vi "Calculate And Insert Biometry State.vi"(8 "error in (no error)":errorcluster caption="错误输入（无错误）", 10 "Measure_No":i64, 11 "connection reference":T1) -> (0 "error out":errorcluster caption="错误输出")   [LabVIEW 2015, in "Boimetry Processing.lvlib"]
doc: "对当初测量第几次的所有测试结果进行判断是否正常。\n判断的结果添加到Biometry的State数据库。\n输入：测量的第几次。"
uses:
  Boimetry Processing.lvlib
  <vilib>/addons/database/Connection.llb/Conn ObjectReference.ctl
  Database Processing/Support/Table/Biometry State.ctl
  Database Processing/Database Processing.lvlib
  <vilib>/addons/database/NI_Database_API.lvlib
  <vilib>/Analysis/NI_AALBase.lvlib
panel:
  # "Busy"
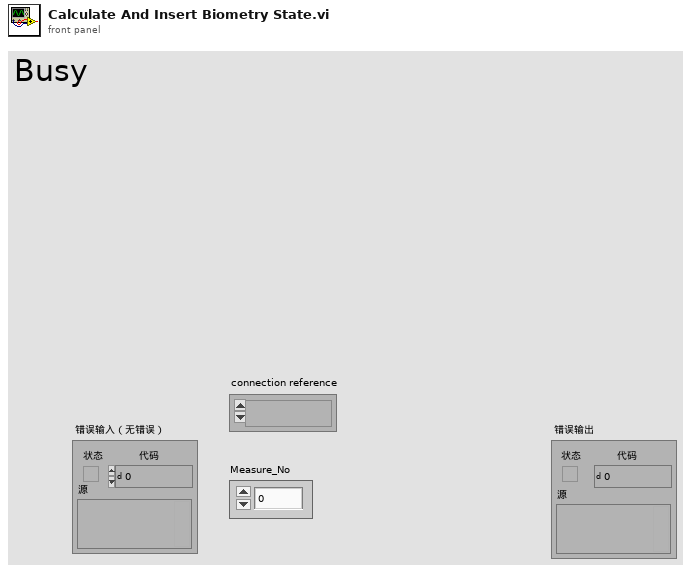
[diagram p1: front panel]
types:
  T1 = typedef "NI_Database_API.lvlib/Conn ObjectReference.ctl" = refnum<k1>
  T2 = typedef "Database Processing.lvlib/Biometry State.ctl" = cluster{"Measure_ID":i64, "Central_Corneal_Thickness_State":string, "Anterior_Chamber_Depth_State":string, "Len_Thickness_State":string, "Retinal_Thickness_State":string, "Axis_Length_State":string, "Pupil_Diameter_State":string, "White_To_White_State":string, "Keratometric_flat_State":string, "Keratometric_steep_State":string}
  T3 = typedef "Database Processing.lvlib/Biometry Attribute.ctl" = cluster{"Measure_ID":i64, "Measure_No":i64, "Ordinal":i64, "L_Or_R":string}
  T4 = typedef "Database Processing.lvlib/Biometry Parameter.ctl" = cluster{"Measure_ID":i64, "Central_Corneal_Thickness":sgl, "Anterior_Chamber_Depth":sgl, "Len_Thickness":sgl, "Retinal_Thickness":sgl, "Axis_Length":sgl, "Pupil_Diameter":sgl, "PCX":sgl, "PCY":sgl, "White_To_White":sgl, "ICX":sgl, "ICY":sgl, "Keratometric_flat":sgl, "Keratometric_steep":sgl, "Keratometric_Axis(flat)":sgl, "Keratometric_Axis(steep)":sgl, "Keratometric_AST":sgl}
  T5 = typedef "Boimetry Processing.lvlib/Limit Configuration.ctl" = cluster{"上限":dbl, "下限":dbl, "误差范围":dbl}[]
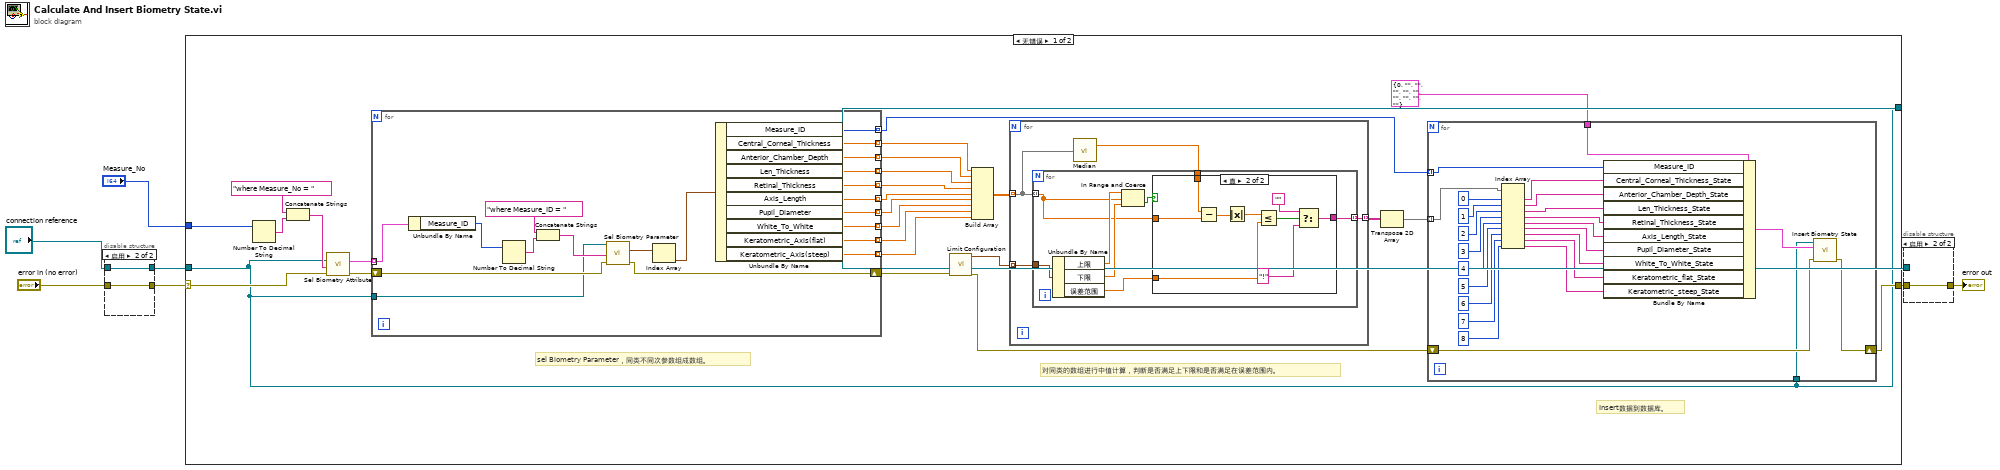
[diagram p0: block diagram]
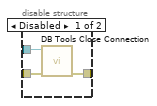
[diagram p2: hidden frame]
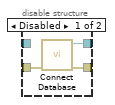
[diagram p3: hidden frame]
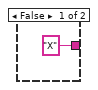
[diagram p4: hidden frame]
diagram:
  n1 = disable-structure shown="启用" {
    disable-tunnel: [w11 w13] -> w8
    disable-tunnel: "error in (no error)" -> [w10 w12]
    disable-tunnel: [w9 w12] -> w6
    disable-tunnel: "connection reference" -> [_ w13]
    frame Disabled {
      n2 = call "Connect Database.vi"("error in (no error)"=w10) -> ("error out"=w9:errorcluster, "connection reference"=w11:T1)  [unwired: 9 in]
    }
    frame Enabled {
    }
  }
  n3 = case shown="无错误" w6 {
    selector: w6 -> [w35 w108]
    tunnel: [w15 w108] -> w4
    tunnel: "Measure_No" -> [w36 _]
    tunnel: w8 -> [w14 w107]
    tunnel: [w14 w107] -> w3
    frame No Error {
      # "Insert数据到数据库。"
      # "对同类的数组进行中值计算，判断是否满足上下限和是否满足在误差范围内。"
      # "sel Biometry Parameter，同类不同次参数组成数组。"
      n4 = Number To Decimal String(number=w36) -> (decimal integer string=w39:string)  [unwired: 1 in]
      n5 = Concatenate Strings("where Measure_No = " ("数据库配置.Condition"), w39) -> (w37:string)
      n6 = call "Sel Biometry Attribute.vi"("error in (no error)"=w35, "condition"=w37, "connection reference"=w14) -> ("error out"=w33:errorcluster, "Biometry Attribute"=w34:T3[])  [unwired: 7 in]
      n7 = for {
        tunnel: w34 -> [w103] mode=indexing
        shift-right: [w88] -> w23
        shift-left: w33 -> [w102]
        tunnel: w14 -> [w100]
        tunnel: [w97] -> w32 mode=indexing
        tunnel: [w96] -> w31 mode=indexing
        tunnel: [w95] -> w30 mode=indexing
        tunnel: [w94] -> w29 mode=indexing
        tunnel: [w93] -> w28 mode=indexing
        tunnel: [w92] -> w27 mode=indexing
        tunnel: [w91] -> w26 mode=indexing
        tunnel: [w90] -> w25 mode=indexing
        tunnel: [w89] -> w24 mode=indexing
        tunnel: [w87] -> w19 mode=indexing
        n8 = Unbundle By Name(w103) -> ("Measure_ID"=w104:i64)
        n9 = Number To Decimal String(number=w104) -> (decimal integer string=w106:string)  [unwired: 1 in]
        n10 = Concatenate Strings("where Measure_ID = " ("数据库配置.Condition"), w106) -> (w101:string)
        n11 = call "Sel Biometry Parameter.vi"("error in (no error)"=w102, "condition"=w101, "connection reference"=w100) -> ("error out"=w88:errorcluster, "Biometry Parameter"=w99:T4[])  [unwired: 7 in]
        n12 = Index Array(array=w99) -> (element=w98:T4)  [unwired: 1 in]
        n13 = Unbundle By Name(w98) -> ("Measure_ID"=w87:i64, "Central_Corneal_Thickness"=w97:sgl, "Anterior_Chamber_Depth"=w96:sgl, "Len_Thickness"=w95:sgl, "Retinal_Thickness"=w94:sgl, "Axis_Length"=w93:sgl, "Pupil_Diameter"=w92:sgl, "White_To_White"=w91:sgl, "Keratometric_Axis(flat)"=w90:sgl, "Keratometric_Axis(steep)"=w89:sgl)
      }
      n14 = call "Limit Configuration.vi"("error in (no error)"=w23) -> ("error out"=w16:errorcluster, "Limit Configuration 2"=w21:T5)  [unwired: 9 in]
      n15 = Build Array(w32, w31, w30, w29, w28, w27, w26, w25, w24) -> (w22:sgl[][])
      n16 = for {
        tunnel: w22 -> [w67] mode=indexing
        tunnel: w21 -> [w68] mode=indexing
        tunnel: [w65] -> w20 mode=indexing
        n17 = call <vilib>:"Median.vi"("X"=w67) -> ("median"=w66:dbl)  [unwired: 1 out]
        n18 = for {
          tunnel: w67 -> [w71] mode=indexing
          tunnel: w68 -> [w76]
          tunnel: w66 -> [w72]
          tunnel: [w69] -> w65 mode=indexing
          n19 = Unbundle By Name(w76) -> ("上限"=w75:dbl, "下限"=w74:dbl, "误差范围"=w70:dbl)
          n20 = In Range and Coerce(upper limit=w75, x=w71, lower limit=w74) -> (In Range?=w73:bool)  [unwired: 1 out]
          n21 = case shown="真" w73 {
            tunnel: w72 -> [_ w86]
            tunnel: w71 -> [_ w85]
            tunnel: w70 -> [_ w82]
            tunnel: ["X" w79] -> w69
            frame False {
            }
            frame True {
              n22 = Subtract(x=w86, y=w85) -> (x-y=w84:dbl)
              n23 = Absolute Value(x=w84) -> (abs(x)=w83:dbl)
              n24 = Less Or Equal?(x=w83, y=w82) -> (x <= y?=w78:bool)
              n25 = Select(t="", s=w78, f="!") -> (s? t:f=w79:string)
            }
          }
        }
      }
      n26 = Transpose 2D Array(2D array=w20) -> (transposed array=w18:string[][])
      n27 = for {
        tunnel: w19 -> [w53] mode=indexing
        tunnel: w18 -> [w55] mode=indexing
        tunnel: T2 {"Measure_ID"=0, "Central_Corneal_Thickness_State"="", "Anterior_Chamber_Depth_State"="", "Len_Thickness_State"="", "Retinal_Thickness_State"="", "Axis_Length_State"="", "Pupil_Diameter_State"="", "White_To_White_State"="", "Keratometric_flat_State"="", "Keratometric_steep_State"=""} ("Biometry State") -> [w54]
        shift-right: [w40] -> w15
        shift-left: w16 -> [w42]
        tunnel: w14 -> [w41]
        n28 = Index Array(array=w55, index #1=0 ("索引"), index #2=1 ("索引"), index #3=2 ("索引"), index #4=3 ("索引"), index #5=4 ("索引"), index #6=5 ("索引"), index #7=6 ("索引"), index #8=7 ("索引"), index #9=8 ("索引")) -> (element #1=w52:string, element #2=w51:string, element #3=w50:string, element #4=w49:string, element #5=w48:string, element #6=w47:string, element #7=w46:string, element #8=w45:string, element #9=w44:string)
        n29 = Bundle By Name(cluster=w54, "Measure_ID"=w53, "Central_Corneal_Thickness_State"=w52, "Anterior_Chamber_Depth_State"=w51, "Len_Thickness_State"=w50, "Retinal_Thickness_State"=w49, "Axis_Length_State"=w48, "Pupil_Diameter_State"=w47, "White_To_White_State"=w46, "Keratometric_flat_State"=w45, "Keratometric_steep_State"=w44) -> (w43:T2)
        n30 = call "Insert Biometry State.vi"("error in (no error)"=w42, "Biometry State"=w43, "connection reference"=w41) -> ("error out"=w40:errorcluster)  [unwired: 8 in]
      }
    }
    frame Error {
    }
  }
  n31 = disable-structure shown="启用" {
    disable-tunnel: w4 -> [w111 w112]
    disable-tunnel: [w110 w112] -> w2
    disable-tunnel: w3 -> [w109 _]
    frame Disabled {
      n32 = call <vilib>:"DB Tools Close Connection.vi"("error in (no error)"=w111, "connection reference"=w109) -> ("error out"=w110:errorcluster)  [unwired: 5 in]
    }
    frame Enabled {
    }
  }
  "error out" <- w2
